vi "Get_Groups_And_Names.vi"(8 "error in (no error)":errorcluster, 10 "Small?":bool, 11 "Constraints":T1 {"Estimate Quality" scale=0.0..5.0}) -> (0 "error out":errorcluster, 1 "Description":string, 2 "Groups":string[](array[string]), 3 "Names":string[](array[string]), 4 "Description Returned?":bool)   [LabVIEW 2013]
doc: "Returns all groups and experiments within the given constraints and (if there is only one group) returns a description of the group and all experiments within the constraints."
uses:
  Controls/Constraints.ctl
  <userlib>/_OpenG.lib/array/array.llb/Remove Duplicates from 1D Array (String)__ogtk.vi
  <userlib>/_OpenG.lib/array/array.llb/Empty 2D Array (Variant)__ogtk.vi
  <vilib>/addons/database/_DB Variant To Data/Database Variant To Data.xnode
panel:
  out "Min-Max experiment settings query":string
  out "Names SQL Query":string
  out "Selected Group":string
  out "Groups SQL Query":string
  out "Description SQL Query":string
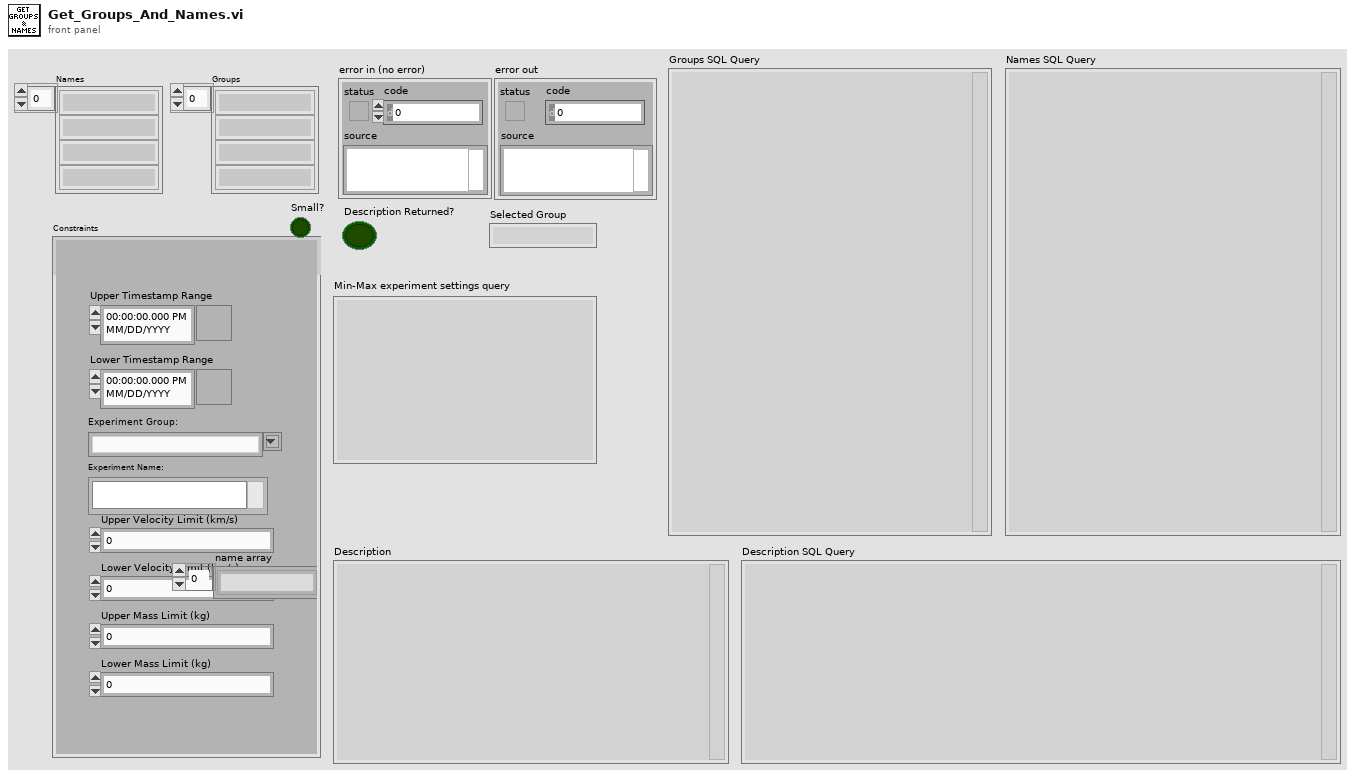
[diagram p1: front panel]
types:
  T1 = typedef "Constraints.ctl" = cluster{"Upper Timestamp Range":timestamp, "Lower Timestamp Range":timestamp, "Experiment Group:":string, "Experiment Name:":i32[], "Upper Velocity Limit (km/s)":dbl, "Lower Velocity Limit (km/s)":dbl, "Upper Mass Limit (kg)":dbl, "Lower Mass Limit (kg)":dbl, "name array":string[], "Estimate Quality":cluster{dbl, dbl}}
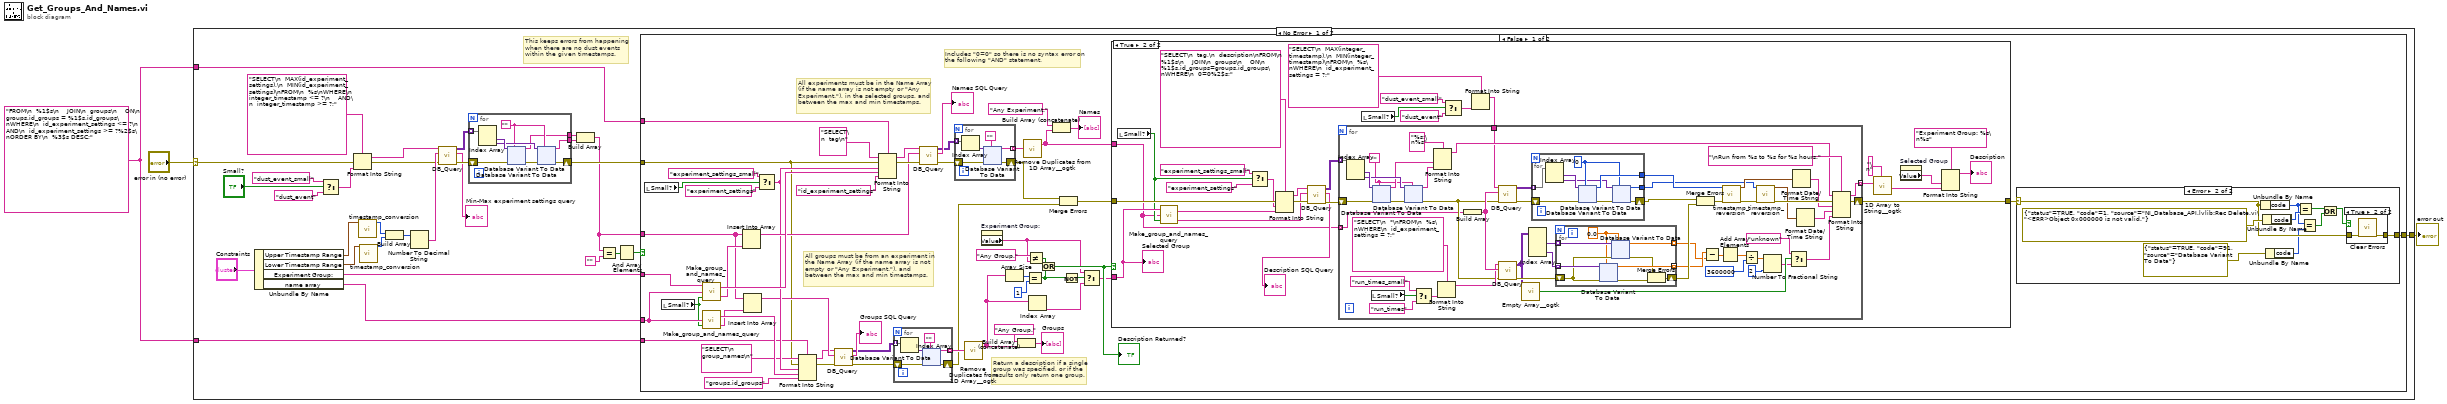
[diagram p0: block diagram]
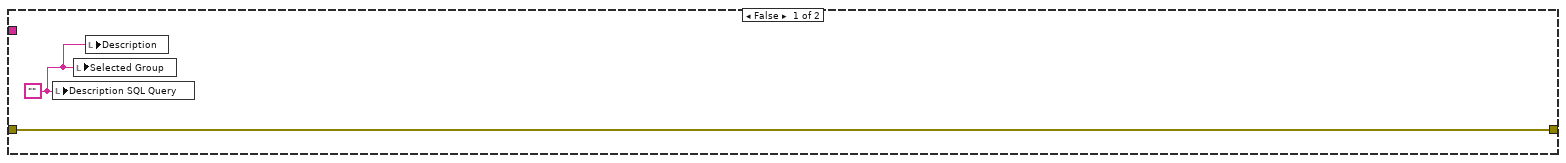
[diagram p4: hidden frame]
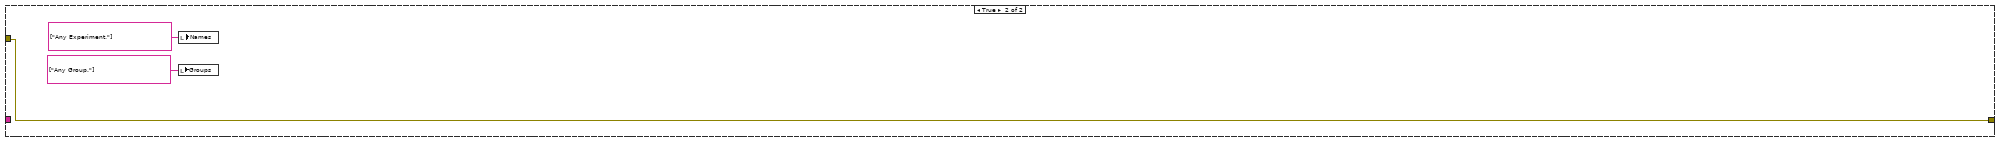
[diagram p5: hidden frame]
diagram:
  w1 = "FROM\n  %1$s\n    JOIN\n  groups\n    ON\n      groups.id_groups = %1$s.id_groups\nWHERE\n  id_experiment_settings <= ?\n    AND\n  id_experiment_settings >= ?%2$s\nORDER BY\n  %3$s DESC;" ("format string")
  n1 = case shown="No Error" "error in (no error)" {
    selector: "error in (no error)" -> [w17 w545]
    tunnel: [w33 w545] -> w3
    tunnel: w1 -> [w22 _]
    tunnel: w1 -> [w21 _]
    frame No Error {
      # "This keeps errors from happening\nwhen there are no dust events\nwithin the given timestamps."
      n2 = Unbundle By Name("Constraints") -> ("Upper Timestamp Range"=w31:timestamp, "Lower Timestamp Range"=w32:timestamp, "Experiment Group:"=w20:string, "name array"=w29:string[])
      n3 = Select(t="dust_event_small", s="Small?", f="dust_event") -> (s? t:f=w18:string)
      n4 = Format Into String(format string="SELECT\n  MAX(id_experiment_settings),\n  MIN(id_experiment_settings)\nFROM\n  %s\nWHERE\n  integer_timestamp <= ?\n    AND\n  integer_timestamp >= ?;", error in=w17, w18) -> (resulting string=w15:string, error out=w14:errorcluster)  [unwired: 1 in]
      n5 = call "timestamp_conversion.vi"("Time Stamp"=w31) -> ("Integer Time"=w26:i64)  [unwired: 8 in, 1 out]
      n6 = call "timestamp_conversion.vi"("Time Stamp"=w32) -> ("Integer Time"=w25:i64)  [unwired: 8 in, 1 out]
      n7 = Build Array(w26, w25) -> (w24:i64[])
      n8 = Number To Decimal String(number=w24) -> (decimal integer string=w16:string[])  [unwired: 1 in]
      n9 = call "DB_Query.vi"("error in (no error)"=w14, "Parameters"=w16, "Parameterized Query"=w15) -> ("error out"=w13:errorcluster, "Query in Standard Format"=→"Min-Max experiment settings query":string, "Results"=w12:variant[][])  [unwired: 6 in]
      n10 = for {
        shift-right: [w474] -> w11
        shift-left: w13 -> [w479]
        tunnel: w12 -> [w480] mode=indexing
        tunnel: [w473] -> w10
        tunnel: [w472] -> w9
        w475 = "" ("t")
        n11 = Index Array(array=w480) -> (element #1=w478:variant, element #2=w476:variant)  [unwired: 2 in]
        n12 = xnode "Database Variant To Data"("database variant"=w478, "error in (no error)"=w479, "type"=w475) -> ("data"=w473:string, "error out"=w477:errorcluster)
        n13 = xnode "Database Variant To Data"("database variant"=w476, "error in (no error)"=w477, "type"=w475) -> ("data"=w472:string, "error out"=w474:errorcluster)
      }
      n14 = Build Array(w10, w9) -> (w7:string[])
      n15 = Equal?(x=w7, y="") -> (x = y?=w4:bool[])
      n16 = And Array Elements(Boolean array=w4) -> (logical AND=w5:bool)
      n17 = case shown="False" w5 {
        tunnel: [w87 w471] -> w33
        tunnel: w29 -> [w66 _]
        tunnel: w22 -> [w41 _]
        tunnel: w21 -> [w40 _]
        tunnel: w20 -> [w39 _]
        tunnel: w11 -> [w35 w471]
        tunnel: w7 -> [w34 _]
        frame False {
          # "Includes \"0=0\" so there is no syntax error on\nthe following \"AND\" statement."
          # "Return a description if a single\ngroup was specified, or if the\nresults only return one group."
          # "All groups must be from an experiment in\nthe Name Array (if the name array is not\nempty or \"Any Experiment.\"), and\nbetween the max and min timestamps."
          # "All experiments must be in the Name Array\n(if the name array is not empty or \"Any\nExperiment.\"), in the selected groups, and\nbetween the max and min timestamps."
          n18 = local read "Small?"() -> (w36:bool)
          n19 = local read "Small?"() -> (w37:bool)
          n20 = call "Make_group_and_names_query.vi"("Small?"=w37, "Name Array"=w66) -> ("Parameters"=w53:string[], "Group and Names Query"=w54:string)  [unwired: 1 in]
          n21 = call "Make_group_and_names_query.vi"("Small?"=w37, "Name Array"=w66, "Group  Name"=w39) -> ("Parameters"=w60:string[], "Group and Names Query"=w63:string)
          n22 = Insert Into Array(array=w34, new element=w60) -> (w57:string[])  [unwired: 1 in]
          n23 = Insert Into Array(array=w34, new element=w53) -> (w51:string[])  [unwired: 1 in]
          n24 = Select(t="experiment_settings_small", s=w36, f="experiment_settings") -> (s? t:f=w55:string)
          n25 = Format Into String(format string=w40, initial string="SELECT\n  group_names\n", error in=w35, w55, w54, "groups.id_groups" ("input 4")) -> (resulting string=w50:string, error out=w52:errorcluster)
          n26 = call "DB_Query.vi"("error in (no error)"=w52, "Parameters"=w51, "Parameterized Query"=w50) -> ("error out"=w47:errorcluster, "Query in Standard Format"=→"Groups SQL Query":string, "Results"=w48:variant[][])  [unwired: 6 in]
          n27 = Format Into String(format string=w41, initial string="SELECT\n  tag\n", error in=w35, w55, w63, "id_experiment_settings" ("input 4")) -> (resulting string=w62:string, error out=w61:errorcluster)
          n28 = for {
            tunnel: [w433] -> w84 mode=indexing
            shift-right: [w432] -> w81
            shift-left: w47 -> [w436]
            tunnel: w48 -> [w431] mode=indexing
            n29 = Index Array(array=w431) -> (element=w434:variant)  [unwired: 1 in]
            n30 = xnode "Database Variant To Data"("database variant"=w434, "error in (no error)"=w436, "type"="" ("t")) -> ("data"=w433:string, "error out"=w432:errorcluster)
          }
          n31 = call "DB_Query.vi"("error in (no error)"=w61, "Parameters"=w57, "Parameterized Query"=w62) -> ("error out"=w56:errorcluster, "Query in Standard Format"=→"Names SQL Query":string, "Results"=w58:variant[][])  [unwired: 6 in]
          n32 = for {
            tunnel: [w89] -> w85 mode=indexing
            shift-right: [w90] -> w82
            shift-left: w56 -> [w93]
            tunnel: w58 -> [w88] mode=indexing
            n33 = Index Array(array=w88) -> (element=w91:variant)  [unwired: 1 in]
            n34 = xnode "Database Variant To Data"("database variant"=w91, "error in (no error)"=w93, "type"="" ("t")) -> ("data"=w89:string, "error out"=w90:errorcluster)
          }
          n35 = call-poly <userlib>:"Remove Duplicates from 1D Array__ogtk.vi"("Input Array"=w84) -> ("Output Array"=w70:string[])  [unwired: 1 out]
          n36 = property on="Experiment Group:" class="CmbBox"() -> ("Value"=w38:string)  [unwired: 2 in, 2 out]
          n37 = Array Size(array=w70) -> (size(s)=w78:i32)
          n38 = Build Array (concatenate)("Any Group.", w70) -> (→"Groups":string[])
          n39 = call-poly <userlib>:"Remove Duplicates from 1D Array__ogtk.vi"("Input Array"=w85) -> ("Output Array"=w46:string[])  [unwired: 1 out]
          n40 = Equal?(x=w78, y=1) -> (x = y?=w71:bool)
          n41 = Not Equal?(x="Any Group.", y=w38) -> (x != y?=w74:bool)
          n42 = Index Array(array=w70) -> (element=w69:string)  [unwired: 1 in]
          n43 = Or(x=w74, y=w71) -> (x .or. y?=w72:bool)
          "Description Returned?" <- w72
          n44 = Build Array (concatenate)("Any Experiment.", w46) -> (→"Names":string[])
          n45 = Merge Errors(w82, w81) -> (w80:errorcluster)
          n46 = Not(x=w71) -> (.not. x?=w67:bool)
          n47 = Select(t=w38, s=w67, f=w69) -> (s? t:f=w68:string)
          n48 = case shown="True" w72 {
            tunnel: w80 -> [w141 w169]
            tunnel: [w141 w168] -> w79
            tunnel: w46 -> [_ w142]
            tunnel: w68 -> [_ w164]
            frame False {
              w140 = ""
              n49 = local write "Description SQL Query"(w140) -> ()
              n50 = local write "Selected Group"(w140) -> ()
              n51 = local write "Description"(w140) -> ()
            }
            frame True {
              n52 = local read "Small?"() -> (w160:bool)
              n53 = call "Make_group_and_names_query.vi"("Small?"=w160, "Name Array"=w142, "Group  Name"=w164) -> ("Parameters"=w156:string[], "Group and Names Query"=w163:string)
              n54 = Select(t="experiment_settings_small", s=w160, f="experiment_settings") -> (s? t:f=w159:string)
              n55 = Format Into String(format string="SELECT\n  tag,\n  description\nFROM\n  %1$s\n    JOIN\n  groups\n    ON\n      %1$s.id_groups=groups.id_groups\nWHERE\n  0=0%2$s;" ("string"), error in=w169, w159, w163) -> (resulting string=w157:string, error out=w158:errorcluster)  [unwired: 1 in]
              n56 = call "DB_Query.vi"("error in (no error)"=w158, "Parameters"=w156, "Parameterized Query"=w157) -> ("error out"=w154:errorcluster, "Query in Standard Format"=→"Description SQL Query":string, "Results"=w155:variant[][])  [unwired: 6 in]
              n57 = local read "Small?"() -> (w148:bool)
              n58 = Select(t="dust_event_small", s=w148, f="dust_event") -> (s? t:f=w147:string)
              n59 = Format Into String(format string="SELECT\n  MAX(integer_timestamp),\n  MIN(integer_timestamp)\nFROM\n  %s\nWHERE\n  id_experiment_settings = ?;", w147) -> (resulting string=w143:string)  [unwired: 2 in, 1 out]
              n60 = for {
                shift-right: [w188] -> w168
                shift-left: w154 -> [w214]
                tunnel: w155 -> [w219] mode=indexing
                tunnel: [w186] -> w152 mode=indexing
                tunnel: w143 -> [w182]
                tunnel: w142 -> [w170] mode=indexing
                w183 = "" ("Integer Time")
                n61 = Index Array(array=w219) -> (element #1=w220:variant, element #2=w218:variant)  [unwired: 2 in]
                n62 = local read "Small?"() -> (w177:bool)
                n63 = xnode "Database Variant To Data"("database variant"=w220, "error in (no error)"=w214, "type"=w183) -> ("data"=w216:string, "error out"=w217:errorcluster)
                n64 = xnode "Database Variant To Data"("database variant"=w218, "error in (no error)"=w217, "type"=w183) -> ("data"=w215:string, "error out"=w171:errorcluster)
                n65 = Select(t="run_times_small", s=w177, f="run_times") -> (s? t:f=w174:string)
                n66 = Format Into String(format string="%s:\n%s", w216, w215) -> (resulting string=w190:string)  [unwired: 2 in, 1 out]
                n67 = Format Into String(format string="SELECT\n  *\nFROM\n  %s\nWHERE\n  id_experiment_settings = ?;", w174) -> (resulting string=w172:string)  [unwired: 2 in, 1 out]
                n68 = Build Array(w170) -> (w181:string[])
                n69 = call "DB_Query.vi"("error in (no error)"=w171, "Parameters"=w181, "Parameterized Query"=w182) -> ("error out"=w180:errorcluster, "Results"=w178:variant[][])  [unwired: 6 in, 1 out]
                n70 = call "DB_Query.vi"("error in (no error)"=w171, "Parameters"=w181, "Parameterized Query"=w172) -> ("error out"=w185:errorcluster, "Results"=w184:variant[][])  [unwired: 6 in, 1 out]
                n71 = call-poly <userlib>:"Empty Array__ogtk.vi"("Array"=w184) -> ("Empty Array?"=w207:bool)  [unwired: 8 in]
                n72 = Index Array(array=w184) -> (element #1=w213:variant[], element #2=w212:variant[])  [unwired: 4 in]
                n73 = for {
                  tunnel: [w228] -> w191
                  shift-right: [w225] -> w200
                  shift-left: w180 -> [w227]
                  tunnel: [w222] -> w179
                  tunnel: w178 -> [w221] mode=indexing
                  w224 = i64 0
                  n74 = Index Array(array=w221) -> (element #1=w229:variant, element #2=w223:variant)  [unwired: 2 in]
                  n75 = xnode "Database Variant To Data"("database variant"=w229, "error in (no error)"=w227, "type"=w224) -> ("data"=w228:i64, "error out"=w226:errorcluster)
                  n76 = xnode "Database Variant To Data"("database variant"=w223, "error in (no error)"=w226, "type"=w224) -> ("data"=w222:i64, "error out"=w225:errorcluster)
                }
                n77 = for {
                  tunnel: w213 -> [w302] mode=indexing
                  tunnel: w212 -> [w301] mode=indexing
                  tunnel: [w298] -> w203 mode=indexing
                  tunnel: [w300] -> w202 mode=indexing
                  shift-right: [w295] -> w204
                  shift-left: w185 -> [w299]
                  w294 = 0.0
                  n78 = xnode "Database Variant To Data"("database variant"=w301, "error in (no error)"=w299, "type"=w294) -> ("data"=w298:dbl, "error out"=w296:errorcluster)
                  n79 = xnode "Database Variant To Data"("database variant"=w302, "error in (no error)"=w299, "type"=w294) -> ("data"=w300:dbl, "error out"=w297:errorcluster)
                  n80 = Merge Errors(w297, w296) -> (w295:errorcluster)
                }
                n81 = Merge Errors(w200, w204) -> (w189:errorcluster)
                n82 = Subtract(x=w203, y=w202) -> (x-y=w201:dbl[])
                n83 = Add Array Elements(numeric array=w201) -> (sum=w211:dbl)
                n84 = call "timestamp_reversion.vi"("error in (no error)"=w189, "Integer Timestamp"=w191) -> ("error out"=w193:errorcluster, "time stamp"=w195:timestamp)  [unwired: 7 in]
                n85 = Divide(x=w211, y=i64 3600000) -> (x/y=w209:dbl)
                n86 = call "timestamp_reversion.vi"("error in (no error)"=w193, "Integer Timestamp"=w179) -> ("error out"=w199:errorcluster, "time stamp"=w194:timestamp)  [unwired: 7 in]
                n87 = Number To Fractional String(number=w209, precision (6)=i16 2) -> (F-format string=w206:string)  [unwired: 2 in]
                n88 = Select(t="unknown" ("f"), s=w207, f=w206) -> (s? t:f=w192:string)
                n89 = Format Date/Time String(seconds (now)=w195) -> (date/time string=w197:string)  [unwired: 2 in]
                n90 = Format Date/Time String(seconds (now)=w194) -> (date/time string=w198:string)  [unwired: 2 in]
                n91 = Format Into String(format string="\nRun from %s to %s for %s hours.", initial string=w190, error in=w199, w197, w198, w192) -> (resulting string=w186:string, error out=w188:errorcluster)
              }
              n92 = call <userlib>:"1D Array to String__ogtk.vi"("delimiter (Tab)"="\n", "Array of Strings"=w152) -> ("delimited string"=w151:string)  [unwired: 9 in]
              n93 = property on="Selected Group" class="Str"() -> ("Value"=w166:string)  [unwired: 2 in, 2 out]
              n94 = Format Into String(format string="Experiment Group: %s\n%s", w166, w151) -> (resulting string=→"Description":string)  [unwired: 2 in, 1 out]
              "Selected Group" <- w164
            }
          }
          n95 = case shown="Error" w79 {
            selector: w79 -> [w126 w133]
            tunnel: [w126 w134] -> w87
            frame No Error {
            }
            frame Error {
              n96 = Unbundle By Name(w133) -> ("code"=w128:i32)
              n97 = Unbundle By Name(errorcluster {"status"=TRUE, "code"=1, "source"="NI_Database_API.lvlib:Rec Delete.vi\"<ERR>Object 0x000000 is not valid."} ("error out")) -> ("code"=w135:i32)
              n98 = Unbundle By Name(errorcluster {"status"=TRUE, "code"=91, "source"="Database Variant To Data"} ("error out")) -> ("code"=w127:i32)
              n99 = Equal?(x=w128, y=w135) -> (x = y?=w131:bool)
              n100 = Equal?(x=w128, y=w127) -> (x = y?=w129:bool)
              n101 = Or(x=w131, y=w129) -> (x .or. y?=w130:bool)
              n102 = case shown="True" w130 {
                tunnel: [w137 w138] -> w134
                tunnel: w133 -> [w137 w139]
                frame False {
                }
                frame True {
                  n103 = call <vilib>:"Clear Errors.vi"("error in (no error)"=w139) -> ("error out"=w138:errorcluster)  [unwired: 6 in]
                }
              }
            }
          }
        }
        frame True {
          n104 = local write "Groups"(string[] ["Any Group."] ("Names")) -> ()
          n105 = local write "Names"(string[] ["Any Experiment."] ("Names")) -> ()
        }
      }
    }
    frame Error {
    }
  }
  "error out" <- w3
